vi "array to data claster.vi"(11 "Array":u64[](array[numeric])) -> (3 "Cluster":T1={"PW"=0, "frequency shift"=0.0, "amp"=0.9999923706054688, "mode type"=0, "mode file"=0, "mode depth"=0, "filter rate_pulse"=0, "filter rate bpsk"=0})   [LabVIEW 2021]
doc: "convert compresed data to PDW for the DDS"
uses:
  pdw.ctl
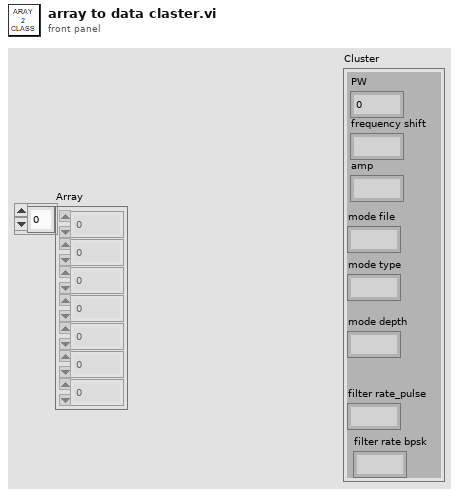
[diagram p1: front panel]
types:
  T1 = typedef "pdw.ctl" = cluster{"PW":u32, "frequency shift":fxp<+/-,48,0>, "amp":fxp<+/-,18,1>, "mode type":u8, "mode file":u8, "mode depth":u32, "filter rate_pulse":u16, "filter rate bpsk":u16}
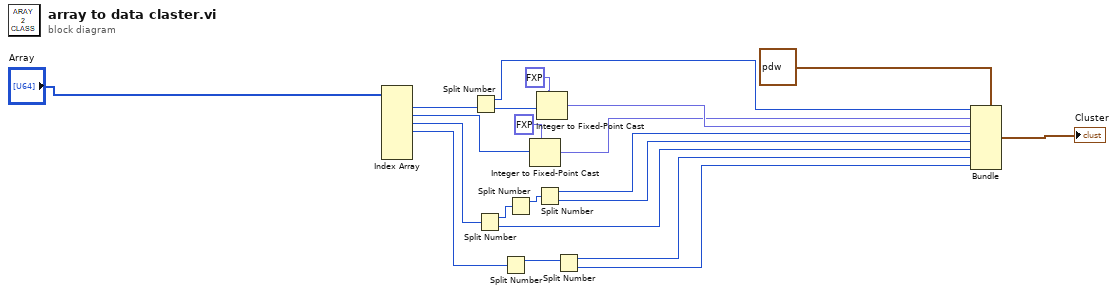
[diagram p0: block diagram]
diagram:
  n1 = Index Array(array="Array") -> (element #1=w17:u64, element #2=w19:u64, element #3=w8:u64, element #4=w4:u64)  [unwired: 7 in, 3 out]
  n2 = Split Number(x=w17) -> (hi(x)=w13:u32, lo(x)=w21:u32)
  n3 = Split Number(x=w8) -> (hi(x)=w10:u32, lo(x)=w5:u32)
  n4 = Split Number(x=w4) -> (hi(x)=w3:u32)  [unwired: 1 out]
  n5 = Split Number(x=w10) -> (hi(x)=w9:u16)  [unwired: 1 out]
  n6 = Integer to Fixed-Point Cast(fixed-point type=fxp<+/-,48,0> 0.0 ("frequency shift"), integer=w19) -> (fixed-point=w11:fxp<+/-,48,0>)
  n7 = Split Number(x=w9) -> (hi(x)=w7:u8, lo(x)=w6:u8)
  n8 = Integer to Fixed-Point Cast(fixed-point type=fxp<+/-,18,1> 0.0 ("I"), integer=w21) -> (fixed-point=w12:fxp<+/-,18,1>)
  n9 = Split Number(x=w3) -> (hi(x)=w2:u16, lo(x)=w1:u16)
  n10 = Bundle(cluster=T1 {"PW"=0, "frequency shift"=0.0, "amp"=0.9999923706054688, "mode type"=0, "mode file"=0, "mode depth"=0, "filter rate_pulse"=0, "filter rate bpsk"=0} ("Cluster"), "PW"=w13, "frequency shift"=w11, "amp"=w12, "mode type"=w7, "mode file"=w6, "mode depth"=w5, "filter rate_pulse"=w2, "filter rate bpsk"=w1) -> (→"Cluster":T1)
